vi "Write.vi"(6 "Append Index":i32, 8 "error in (no error)":errorcluster, 9 "Notes":string, 10 "Data (Dictionary)":T1[](array[typedef]), 11 "Data.ITX in":refnum<class "LV-Data.ITX.lvclass">) -> (0 "error out":errorcluster, 3 "Data.ITX out":refnum<class "LV-Data.ITX.lvclass">, 5 "Path out":path)   [LabVIEW 2019, in "LV-Data.ITX.lvclass"]
uses:
  LV-Data.ITX.lvclass
  C:/Users/patrick/Documents/GitHub/LV-Data/src/LV-Data/LV-Data.lvclass
  LV-Data/Typedefs/Dictionary--cluster.ctl
  LV-Data/LV-Data.lvclass/LV-Data.ctl
  LV-Data.ITX.lvclass/LV-Data.ITX.ctl
  30809772-43d8-4a24-8c66-b05407d0e833.vi
  30809772-43d8-4a24-8c66-b05407d0e833.vi/5de7d03b-c574-4570-ab0d-6535f7e4a6b1.vi
  30809772-43d8-4a24-8c66-b05407d0e833.vi/2d4a6ce1-3f9a-4f39-94c1-e2720b9899a8.vi
  <vilib>/AdvancedString/1D String Array to Delimited String.vi
  private/Variant to ITX Wave.vi
  private/Commands to ITX.vi
  private/Notes to ITX.vi
  LV-Data/LV-Data.lvclass
  ITX Commands/ITX Commands.lvclass
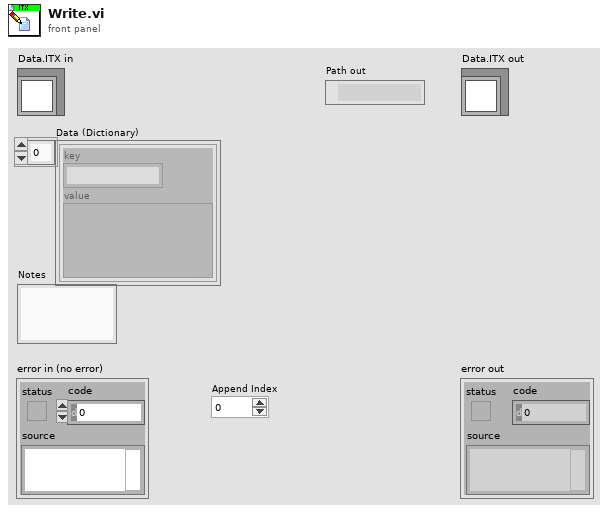
[diagram p1: front panel]
types:
  T1 = typedef "LV-Data.lvclass/Dictionary--cluster.ctl" = cluster{"key":string, "value":variant}
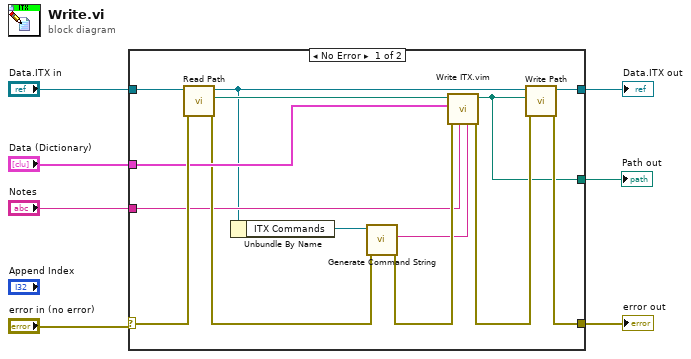
[diagram p0: block diagram]
diagram:
  n1 = case shown="No Error" "error in (no error)" {
    selector: "error in (no error)" -> [w20 w23]
    tunnel: [w18 w23] -> w4
    tunnel: "Data.ITX in" -> [w21 w22]
    tunnel: [w19 w22] -> w5
    tunnel: "Data (Dictionary)" -> [w16 _]
    tunnel: "Notes" -> [w9 _]
    tunnel: [w11 _] -> w1
    frame No Error {
      n2 = call "Read Path.vi"("error in (no error)"=w20, "Data Save"=w21) -> ("error out"=w14:errorcluster, "Path"=w12:path, "Data Save out"=w8:refnum<class "LV-Data.ITX.lvclass">)  [unwired: 7 in]
      n3 = Unbundle By Name(w8) -> ("ITX Commands"=w15:refnum<class "ITX Commands.lvclass">)
      n4 = call "Generate Command String.vi"("ITX Commands in"=w15, "error in (no error)"=w14) -> ("ITX Commands"=w10:string, "error out"=w13:errorcluster)  [unwired: 6 in, 1 out]
      n5 = call "Write ITX.vim"("commands"=w10, "notes"=w9, "error in"=w13, "values"=w16, "filename"=w12) -> ("error out"=w17:errorcluster, "filename out"=w11:path)  [unwired: 4 in, 1 out]
      n6 = call "Write Path.vi"("error in (no error)"=w17, "Path"=w11, "Data Save"=w8) -> ("error out"=w18:errorcluster, "Data Save out"=w19:refnum<class "LV-Data.ITX.lvclass">)  [unwired: 7 in]
    }
    frame Error {
    }
  }
  "error out" <- w4
  "Data.ITX out" <- w5
  "Path out" <- w1
